vi "GrayToRGB.vi"() -> ()   [LabVIEW 2019]
uses:
  GrayToRGBAlternative DLL Project/VI Project/GrayToRGBAlternative.dll
panel:
  in  "Available Colormaps":T1
  out "RGB Image":T2(plugin-control)
  out "Elapsed Time in C (sec)":dbl
  out "Gray Image":T2(plugin-control)
  in  "Gray Image Path":path
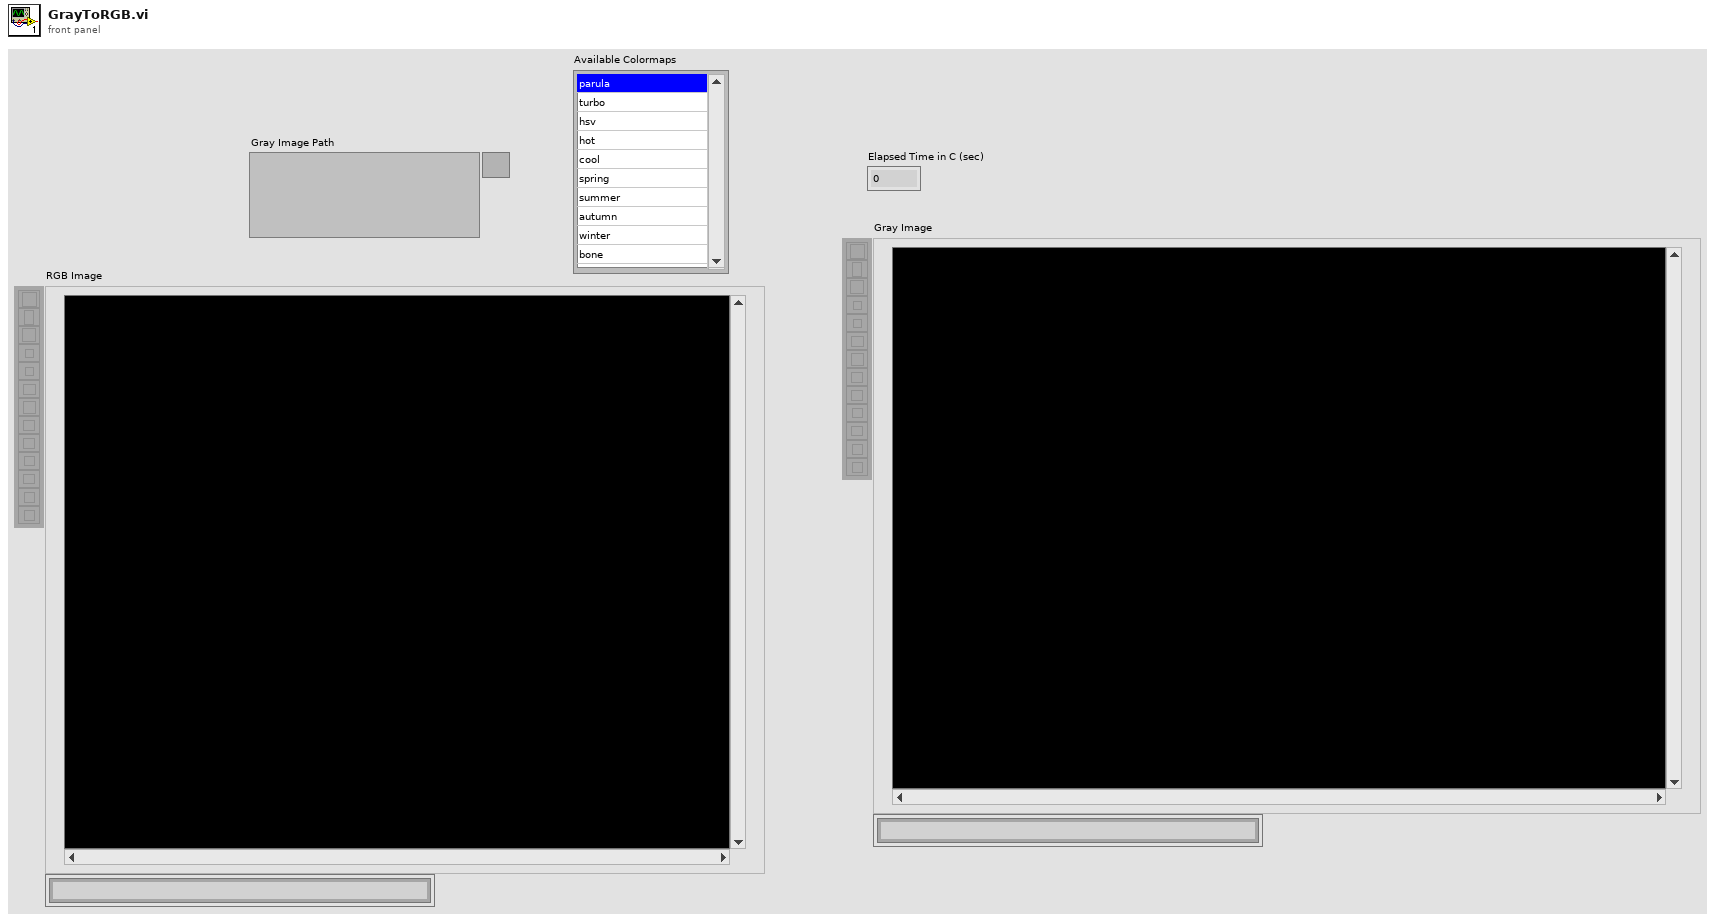
[diagram p1: front panel]
types:
  T1 = typedef "Control 1.ctl" = i32
  T2 = typedef "IMAQ Image.ctl" = refnum<image>
  T3 = enum32{"Map Pixel Pointer", "Unmap Pixel Pointer", "Get Pixels Infos"}
  T4 = typedef "Image Type" = u32
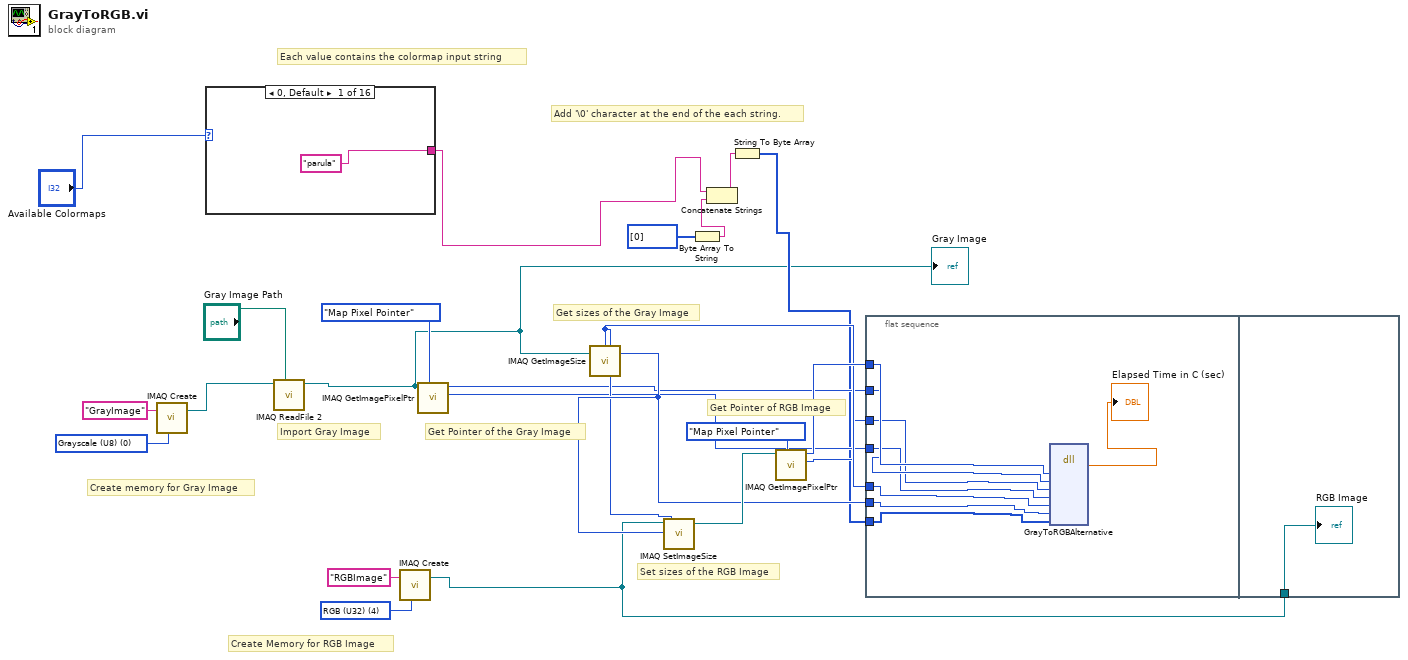
[diagram p0: block diagram]
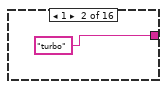
[diagram p2: hidden frame]
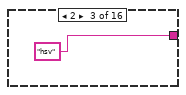
[diagram p3: hidden frame]
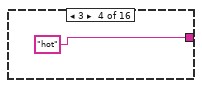
[diagram p4: hidden frame]
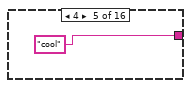
[diagram p5: hidden frame]
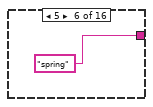
[diagram p6: hidden frame]
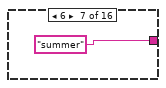
[diagram p7: hidden frame]
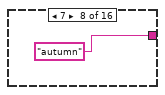
[diagram p8: hidden frame]
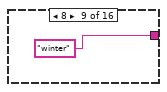
[diagram p9: hidden frame]
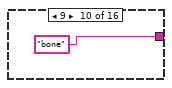
[diagram p10: hidden frame]
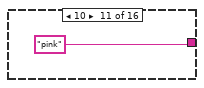
[diagram p11: hidden frame]
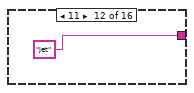
[diagram p12: hidden frame]
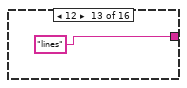
[diagram p13: hidden frame]
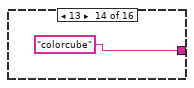
[diagram p14: hidden frame]
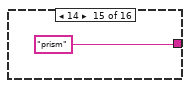
[diagram p15: hidden frame]
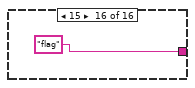
[diagram p16: hidden frame]
diagram:
  w17 = T4 4 items=["Grayscale (U8)", "Grayscale (I16)", "Grayscale (SGL)", "Complex (CSG)", "RGB (U32)", "HSL (U32)", "RGB (U64)", "Grayscale (U16)"] ("Image Type")
  w21 = T4 0 items=["Grayscale (U8)", "Grayscale (I16)", "Grayscale (SGL)", "Complex (CSG)", "RGB (U32)", "HSL (U32)", "RGB (U64)", "Grayscale (U16)"] ("Image Type")
  # "Each value contains the colormap input string"
  # "Get Pointer of RGB Image"
  # "Set sizes of the RGB Image"
  # "Create Memory for RGB Image"
  # "Get sizes of the Gray Image"
  # "Get Pointer of the Gray Image"
  # "Import Gray Image"
  # "Create memory for Gray Image"
  # "Add '\\0' character at the end of the each string."
  n1 = call "IMAQ Create"("Image Name"="GrayImage", "Image Type"=w21) -> ("New Image"=w20:T2)  [unwired: 3 in, 1 out]
  n2 = case shown="0, Default" "Available Colormaps" {
    tunnel: ["parula" "turbo" "hsv" "hot" "cool" "spring" "summer" "autumn" "winter" "bone" "pink" "jet" "lines" "colorcube" "prism" "flag"] -> w5
    frame 0, Default {
    }
    frame 1 {
    }
    frame 2 {
    }
    frame 3 {
    }
    frame 4 {
    }
    frame 5 {
    }
    frame 6 {
    }
    frame 7 {
    }
    frame 8 {
    }
    frame 9 {
    }
    frame 10 {
    }
    frame 11 {
    }
    frame 12 {
    }
    frame 13 {
    }
    frame 14 {
    }
    frame 15 {
    }
  }
  n3 = call "IMAQ ReadFile 2"("File Path"="Gray Image Path", "Image"=w20) -> ("Image Out"=w1:T2)  [unwired: 5 in, 4 out]
  "Gray Image" <- w1
  n4 = call "IMAQ Create"("Image Name"="RGBImage", "Image Type"=w17) -> ("New Image"=w2:T2)  [unwired: 3 in, 1 out]
  n5 = call "IMAQ GetImagePixelPtr"("Function"=T3."Map Pixel Pointer", "Image"=w1) -> ("LineWidth(Pixels)"=w10:i32, "Pixel Pointer out"=w11:u64)  [unwired: 4 in, 4 out]
  n6 = call "IMAQ GetImageSize"("Image"=w1) -> ("Y Resolution"=w14:i32, "X Resolution"=w12:i32)  [unwired: 3 in, 1 out]
  n7 = call "IMAQ SetImageSize"("Y Resolution"=w14, "X Resolution"=w12, "Image"=w2) -> ("Image Out"=w16:T2)  [unwired: 2 in, 1 out]
  n8 = Byte Array To String(unsigned byte array=u8[] [0]) -> (string=w4:string)
  n9 = Concatenate Strings(w5, w4) -> (w3:string)
  n10 = String To Byte Array(string=w3) -> (unsigned byte array=w8:u8[])
  n11 = call "IMAQ GetImagePixelPtr"("Function"=T3."Map Pixel Pointer", "Image"=w16) -> ("LineWidth(Pixels)"=w9:i32, "Pixel Pointer out"=w13:u64)  [unwired: 4 in, 4 out]
  n12 = flat-sequence {
    tunnel: w14 -> [w42]
    tunnel: w12 -> [w43]
    tunnel: w13 -> [w47]
    tunnel: w11 -> [w46]
    tunnel: w10 -> [w44]
    tunnel: w9 -> [w45]
    tunnel: w8 -> [w41]
    tunnel: w2 -> [w48]
    frame #0 {
      n13 = dll-call lib="C:/Users/byald/Desktop/EE-433 Project Group1/GrayToRGBAlternative DLL Project/VI Project/GrayToRGBAlternative.dll" fn="GrayToRGBAlternative"("RGBImage"=w47, "GrayImage"=w46, "LVLineWidthRGB"=w45, "LVLineWidthGray"=w44, "LVWidth"=w43, "LVHeight"=w42, "ColorMap"=w41) -> ("return type"=→"Elapsed Time in C (sec)":dbl)  [unwired: 10 in, 2 out]
    }
    frame #1 {
      "RGB Image" <- w48
    }
  }
